vi "Set Counter Prefix.vi"(8 "error in":errorcluster, 11 "counter interface in":refnum<class "Counter Interface.lvclass">) -> (0 "error out":errorcluster, 3 "counter interface out":refnum<class "Counter Interface.lvclass">)   [LabVIEW 2017, in "Counter Interface.lvclass"]
uses:
  Counter Interface.lvclass
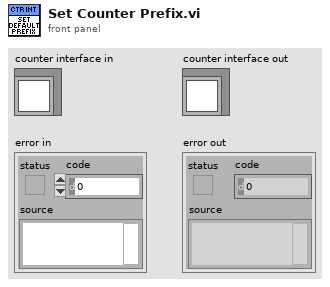
[diagram p1: front panel]
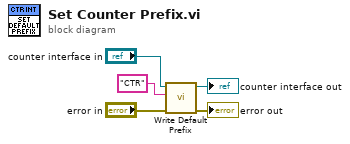
[diagram p0: block diagram]
diagram:
  n1 = call-dynamic "Write Default Prefix.vi"("error in"="error in", "default prefix"="CTR" ("Default Prefix"), "channel in"="counter interface in") -> ("error out"=→"error out":errorcluster, "channel out"=→"counter interface out":refnum<class "Counter Interface.lvclass">)  [unwired: 7 in]
